vi "Setcheck.vi"(2 "variablearray":T1(array[cluster])=[{"ling.var."="in1", "x-min"=-1.0, "x-max"=1.0, "setarray"=[{"linguistic term"="NE1", "color"=0, "points"=[-1.0, -1.0, -1.0, 0.0]}, {"linguistic term"="ZE1", "color"=0, "points"=[-1.0, 0.0, 0.0, 1.0]}, {"linguistic term"="PO1", "color"=0, "points"=[0.0, 1.0, 1.0, 1.0]}]}, {"ling.var."="in2", "x-min"=-1.0, "x-max"=1.0, "setarray"=[{"linguistic term"="NE2", "color"=0, "points"=[-1.0, -1.0, -1.0, 0.0]}, {"linguistic term"="ZE2", "color"=0, "points"=[-1.0, 0.0, 0.0, 1.0]}, {"linguistic term"="PO2", "color"=0, "points"=[0.0, 1.0, 1.0, 1.0]}]}, {"ling.var."="in3", "x-min"=-1.0, "x-max"=1.0, "setarray"=[{"linguistic term"="NE3", "color"=0, "points"=[-1.0, -1.0, -1.0, 0.0]}, {"linguistic term"="ZE3", "color"=0, "points"=[-1.0, 0.0, 0.0, 1.0]}, {"linguistic term"="PO3", "color"=0, "points"=[0.0, 1.0, 1.0, 1.0]}]}, {"ling.var."="in4", "x-min"=-1.0, "x-max"=1.0, "setarray"=[{"linguistic term"="NE4", "color"=0, "points"=[-1.0, -1.0, -1.0, 0.0]}, {"linguistic term"="ZE4", "color"=0, "points"=[-1.0, 0.0, 0.0, 1.0]}, {"linguistic term"="PO4", "color"=0, "points"=[0.0, 1.0, 1.0, 1.0]}]}] {"x-min" step=0.009999999776482582 format="%.2f"; "x-max" step=0.009999999776482582 format="%.2f"; "setarray"."points" step=0.009999999776482582 format="%.2f"}) -> (0 "error out":errorcluster)   [LabVIEW 2017, in "NI_fuzzy logic.lvlib"]
doc: "Checks the Setvalues and the range.\nThe VI-Code is the number of the kind of VI. It gives the first two numbers of the errorcode. The second two are given by the kind of error.\n\nError Nr.\na,b,c,d < min ...01\na,b,c,d > max ...02\na>b, b>c, c>d ...03\nMin >= Max ...04"
uses:
  <vilib>/addons/control/fuzzy/NI_fuzzy logic.lvlib
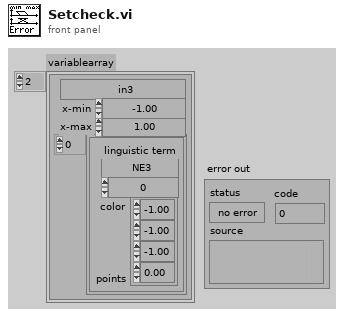
[diagram p1: front panel]
types:
  T1 = cluster{"ling.var.":string, "x-min":dbl, "x-max":dbl, "setarray":cluster{"linguistic term":string, "color":u32, "points":dbl[]}[]}[]
  T2 = cluster{"linguistic term":string, "color":u32, "points":dbl[]}[]
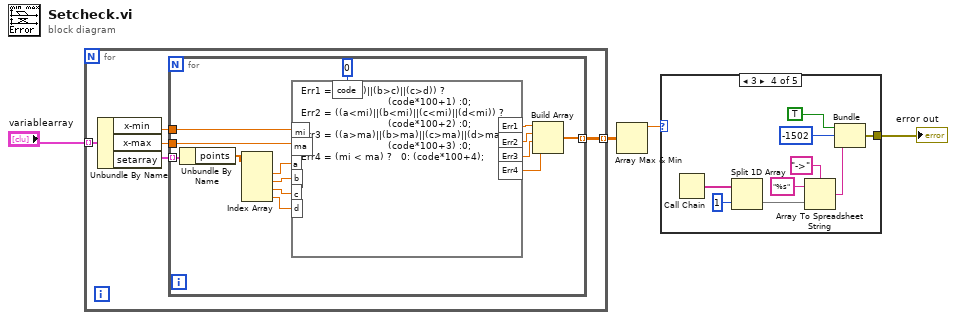
[diagram p0: block diagram]
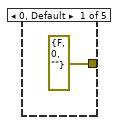
[diagram p2: hidden frame]
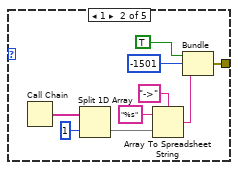
[diagram p3: hidden frame]
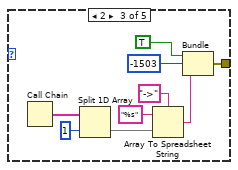
[diagram p4: hidden frame]
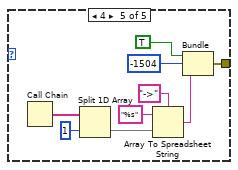
[diagram p5: hidden frame]
diagram:
  n1 = for {
    tunnel: "variablearray" -> [w6] mode=indexing
    tunnel: [w5] -> w3 mode=indexing
    n2 = Unbundle By Name(w6) -> ("x-min"=w9:dbl, "x-max"=w8:dbl, "setarray"=w7:T2)
    n3 = for {
      tunnel: w8 -> [w23]
      tunnel: w9 -> [w22]
      tunnel: w7 -> [w21] mode=indexing
      tunnel: [w10] -> w5 mode=indexing
      n4 = Unbundle By Name(w21) -> ("points"=w19:dbl[])
      n5 = Index Array(array=w19) -> (element #1=w18:dbl, element #2=w15:dbl, element #3=w16:dbl, element #4=w17:dbl)  [unwired: 4 in]
      n6 = formula code="Err1 = ((a>b)||(b>c)||(c>d)) ? \n                             (code*100+1) :0;\nErr2 = ((a<mi)||(b<mi)||(c<mi)||(d<mi)) ?                      \n                             (code*100+2) :0;\nErr3 = ((a>ma)||(b>ma)||(c>ma)||(d>ma))? \n                             (code*100+3) :0;\nErr4 = (mi < ma) ?   0: (code*100+4);"("a"=w18, "b"=w15, "c"=w16, "d"=w17, "mi"=w22, "ma"=w23, "code"=u8 0 ("Input Variable")) -> ("Err1"=w11:dbl, "Err2"=w12:dbl, "Err3"=w13:dbl, "Err4"=w14:dbl)
      n7 = Build Array(w11, w12, w13, w14) -> (w10:dbl[])
    }
  }
  n8 = Array Max & Min(array=w3) -> (max value=w2:dbl)  [unwired: 3 out]
  n9 = case shown="3" w2 {
    tunnel: [cluster{bool, i32, "spreadsheet string":string} {FALSE, 0, "spreadsheet string"=""} w25 w34 w43 w52] -> w1
    frame 0, Default {
    }
    frame 1 {
      n10 = Call Chain() -> (call chain=w29:string[])
      n11 = Split 1D Array(array=w29, index=1) -> (second subarray=w27:string[])  [unwired: 1 out]
      n12 = Array To Spreadsheet String(delimiter (Tab)="->", array=w27, 3:"%s" ("format string")) -> (spreadsheet string=w26:string)
      n13 = Bundle(TRUE, -1501, "spreadsheet string"=w26) -> (w25:cluster{bool, i32, "spreadsheet string":string})  [unwired: 1 out]
    }
    frame 2 {
      n14 = Call Chain() -> (call chain=w38:string[])
      n15 = Split 1D Array(array=w38, index=1) -> (second subarray=w36:string[])  [unwired: 1 out]
      n16 = Array To Spreadsheet String(delimiter (Tab)="->", array=w36, 3:"%s" ("format string")) -> (spreadsheet string=w35:string)
      n17 = Bundle(TRUE, -1503, "spreadsheet string"=w35) -> (w34:cluster{bool, i32, "spreadsheet string":string})  [unwired: 1 out]
    }
    frame 3 {
      n18 = Call Chain() -> (call chain=w47:string[])
      n19 = Split 1D Array(array=w47, index=1) -> (second subarray=w45:string[])  [unwired: 1 out]
      n20 = Array To Spreadsheet String(delimiter (Tab)="->", array=w45, 3:"%s" ("format string")) -> (spreadsheet string=w44:string)
      n21 = Bundle(TRUE, -1502, "spreadsheet string"=w44) -> (w43:cluster{bool, i32, "spreadsheet string":string})  [unwired: 1 out]
    }
    frame 4 {
      n22 = Call Chain() -> (call chain=w56:string[])
      n23 = Split 1D Array(array=w56, index=1) -> (second subarray=w54:string[])  [unwired: 1 out]
      n24 = Array To Spreadsheet String(delimiter (Tab)="->", array=w54, 3:"%s" ("format string")) -> (spreadsheet string=w53:string)
      n25 = Bundle(TRUE, -1504, "spreadsheet string"=w53) -> (w52:cluster{bool, i32, "spreadsheet string":string})  [unwired: 1 out]
    }
  }
  "error out" <- w1
